vi "EPTx_Patch1.0.vi"(6 "Inj_Duration_in":T2, 8 "DrvMode":u32, 9 "Adv_Speed":sgl, 11 "Inj_Timing":T3) -> (4 "Inj_Timing_DBTDC":sgl, 5 "Cmd_Duration":T1 caption="簇")   [LabVIEW 2023]
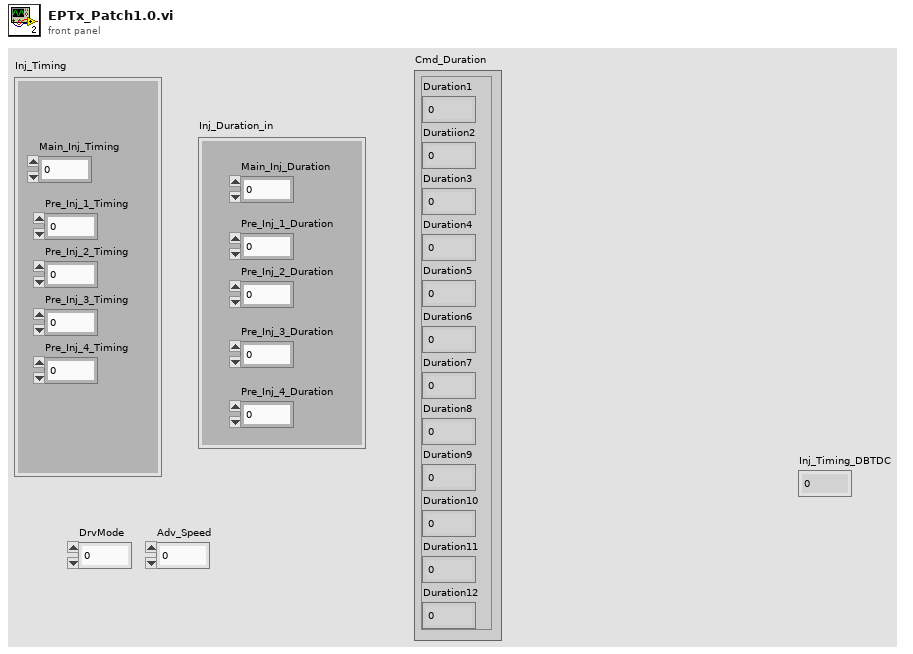
[diagram p1: front panel]
types:
  T1 = cluster{"Duration1":sgl, "Duratiion2":sgl, "Duration3":sgl, "Duration4":sgl, "Duration5":sgl, "Duration6":sgl, "Duration7":sgl, "Duration8":sgl, "Duration9":sgl, "Duration10":sgl, "Duration11":sgl, "Duration12":sgl}
  T2 = cluster{"Main_Inj_Duration":sgl, "Pre_Inj_1_Duration":sgl, "Pre_Inj_2_Duration":sgl, "Pre_Inj_3_Duration":sgl, "Pre_Inj_4_Duration":sgl}
  T3 = cluster{"Main_Inj_Timing":sgl, "Pre_Inj_1_Timing":sgl, "Pre_Inj_2_Timing":sgl, "Pre_Inj_3_Timing":sgl, "Pre_Inj_4_Timing":sgl}
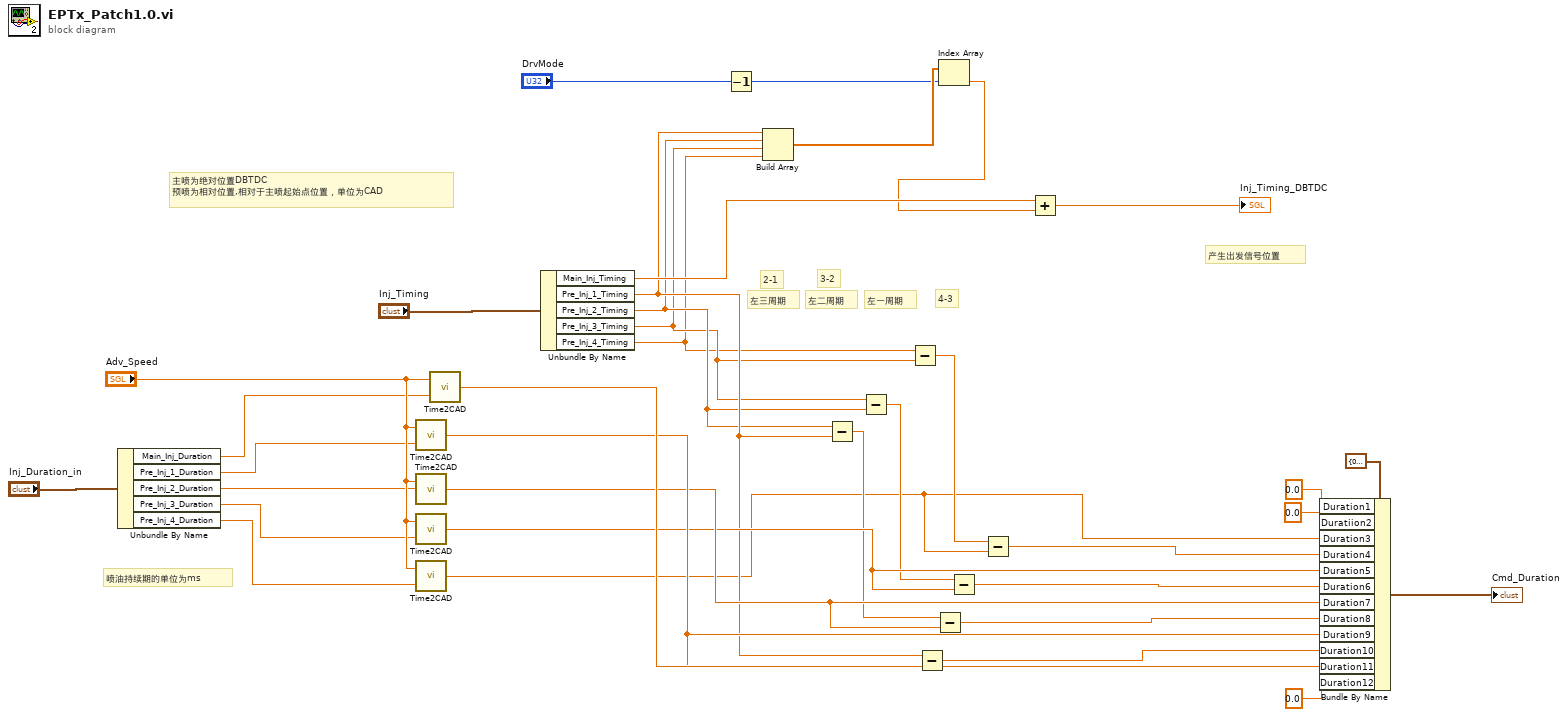
[diagram p0: block diagram]
diagram:
  # "2-1"
  # "3-2"
  # "4-3"
  # "左三周期"
  # "左二周期"
  # "左一周期"
  # "喷油持续期的单位为ms"
  # "产生出发信号位置"
  # "主喷为绝对位置DBTDC\n预喷为相对位置,相对于主喷起始点位置，单位为CAD"
  n1 = Unbundle By Name("Inj_Duration_in") -> ("Main_Inj_Duration"=w28:sgl, "Pre_Inj_1_Duration"=w27:sgl, "Pre_Inj_2_Duration"=w26:sgl, "Pre_Inj_3_Duration"=w25:sgl, "Pre_Inj_4_Duration"=w24:sgl)
  n2 = call <vilib>:"Time2CAD.vi"("Time [ms]"=w27, "Speed (RPM)"="Adv_Speed") -> ("CAD"=w20:sgl)
  n3 = call <vilib>:"Time2CAD.vi"("Time [ms]"=w26, "Speed (RPM)"="Adv_Speed") -> ("CAD"=w18:sgl)
  n4 = call <vilib>:"Time2CAD.vi"("Time [ms]"=w25, "Speed (RPM)"="Adv_Speed") -> ("CAD"=w16:sgl)
  n5 = call <vilib>:"Time2CAD.vi"("Time [ms]"=w24, "Speed (RPM)"="Adv_Speed") -> ("CAD"=w1:sgl)
  n6 = call <vilib>:"Time2CAD.vi"("Time [ms]"=w28, "Speed (RPM)"="Adv_Speed") -> ("CAD"=w22:sgl)
  n7 = Unbundle By Name("Inj_Timing") -> ("Main_Inj_Timing"=w32:sgl, "Pre_Inj_1_Timing"=w9:sgl, "Pre_Inj_2_Timing"=w8:sgl, "Pre_Inj_3_Timing"=w7:sgl, "Pre_Inj_4_Timing"=w6:sgl)
  n8 = Decrement(x="DrvMode") -> (x-1=w2:u32)
  n9 = Build Array(w9, w8, w7, w6) -> (w5:sgl[])
  n10 = Subtract(x=w8, y=w9) -> (x-y=w10:sgl)
  n11 = Subtract(x=w7, y=w8) -> (x-y=w11:sgl)
  n12 = Subtract(x=w6, y=w7) -> (x-y=w12:sgl)
  n13 = Subtract(x=w9, y=w20) -> (x-y=w21:sgl)
  n14 = Subtract(x=w10, y=w18) -> (x-y=w19:sgl)
  n15 = Index Array(array=w5, index=w2) -> (element=w4:sgl)
  n16 = Subtract(x=w11, y=w16) -> (x-y=w17:sgl)
  n17 = Subtract(x=w12, y=w1) -> (x-y=w15:sgl)
  n18 = Add(x=w32, y=w4) -> (x+y=→"Inj_Timing_DBTDC":sgl)
  n19 = Bundle By Name(cluster=T1 {"Duration1"=0.0, "Duratiion2"=0.0, "Duration3"=0.0, "Duration4"=0.0, "Duration5"=0.0, "Duration6"=0.0, "Duration7"=0.0, "Duration8"=0.0, "Duration9"=0.0, "Duration10"=0.0, "Duration11"=0.0, "Duration12"=0.0} ("Cmd_Duration"), "Duration1"=sgl 0.0, "Duratiion2"=sgl 0.0, "Duration3"=w1, "Duration4"=w15, "Duration5"=w16, "Duration6"=w17, "Duration7"=w18, "Duration8"=w19, "Duration9"=w20, "Duration10"=w21, "Duration11"=w22, "Duration12"=sgl 0.0) -> (→"Cmd_Duration":T1)
